vi "end_power_measurements.vi"(7 "Power Meter Connection Data In":T1) -> (15 "error out":errorcluster)   [LabVIEW 2023]
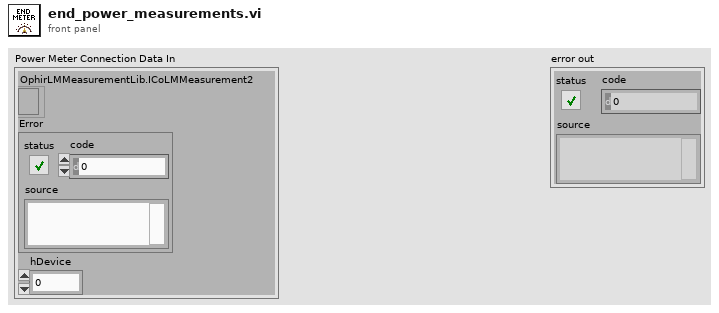
[diagram p1: front panel]
types:
  T1 = cluster{"OphirLMMeasurementLib.ICoLMMeasurement2":refnum<k7>, "Error":errorcluster, "hDevice":i32}
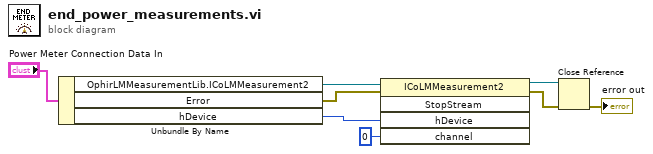
[diagram p0: block diagram]
diagram:
  n1 = Unbundle By Name("Power Meter Connection Data In") -> ("OphirLMMeasurementLib.ICoLMMeasurement2"=w3:refnum<k7>, "Error"=w2:errorcluster, "hDevice"=w1:i32)
  n2 = invoke class="ICoLMMeasurement2" method="StopStream"(reference=w3, error in=w2, "hDevice"=w1, "channel"=0) -> (reference out=w8:refnum<k7>, error out=w7:errorcluster)  [unwired: 1 in, 3 out]
  n3 = Close Reference(reference=w8, error in (no error)=w7) -> (error out=→"error out":errorcluster)
